vi "digital waveforms.vi"(11 "SD method in":T1 {"method array"."offset" format="%.2f"; "method array"."amplitude" format="%.2f"; "method array"."cycles/repeat period" min=1}) -> (2 "waveforms out":T2 format="%.2f", 3 "SD method out":T1 {"method array"."offset" format="%.2f"; "method array"."amplitude" format="%.2f"; "method array"."cycles/repeat period" min=1})   [LabVIEW 2010]
uses:
  SDMethod.ctl
  wavecluster.ctl
  <vilib>/Analysis/NI_AALBase.lvlib
panel:
  # "ticks"
  # "hz"
  # "ticks"
  # "ticks"
  # "volts"
  # "volts"
  # "ticks"
  # "hz"
  # "ticks"
  # "ticks"
  # "volts"
  # "volts"
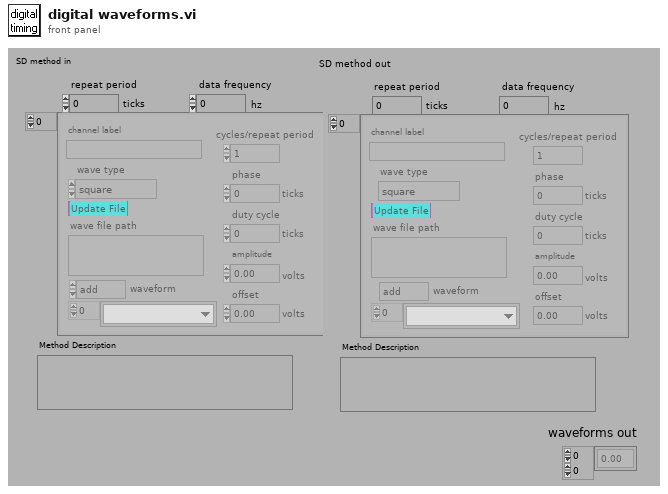
[diagram p1: front panel]
types:
  T1 = typedef "SDMethod.ctl" = cluster{"method array":cluster{"wave type":enum16{"off", "square", "sine", "triangle", "sawtooth", "from file", "wavemaker", "flume pump"}, "cycles/repeat period":u32, "phase":i32, "duty cycle":u32, "wave file path":path, "amplitude":dbl, "channel label":string, "Update":bool, "offset":dbl, " waveform":u16[], "Function":enum16{"add", "multiply"}}[], "Method Description":string, "data frequency":u32, "repeat period":u32}
  T2 = typedef "wavecluster.ctl" = sgl[][]
  T3 = cluster{"wave type":enum16{"off", "square", "sine", "triangle", "sawtooth", "from file", "wavemaker", "flume pump"}, "cycles/repeat period":u32, "phase":i32, "duty cycle":u32, "wave file path":path, "amplitude":dbl, "channel label":string, "Update":bool, "offset":dbl, " waveform":u16[], "Function":enum16{"add", "multiply"}}[]
  T4 = enum16{"off", "square", "sine", "triangle", "sawtooth", "from file", "wavemaker", "flume pump"}
  T5 = cluster{"wave type":enum16{"off", "square", "sine", "triangle", "sawtooth", "from file", "wavemaker", "flume pump"}, "cycles/repeat period":u32, "phase":i32, "duty cycle":u32, "wave file path":path, "amplitude":dbl, "channel label":string, "Update":bool, "offset":dbl, " waveform":u16[], "Function":enum16{"add", "multiply"}}
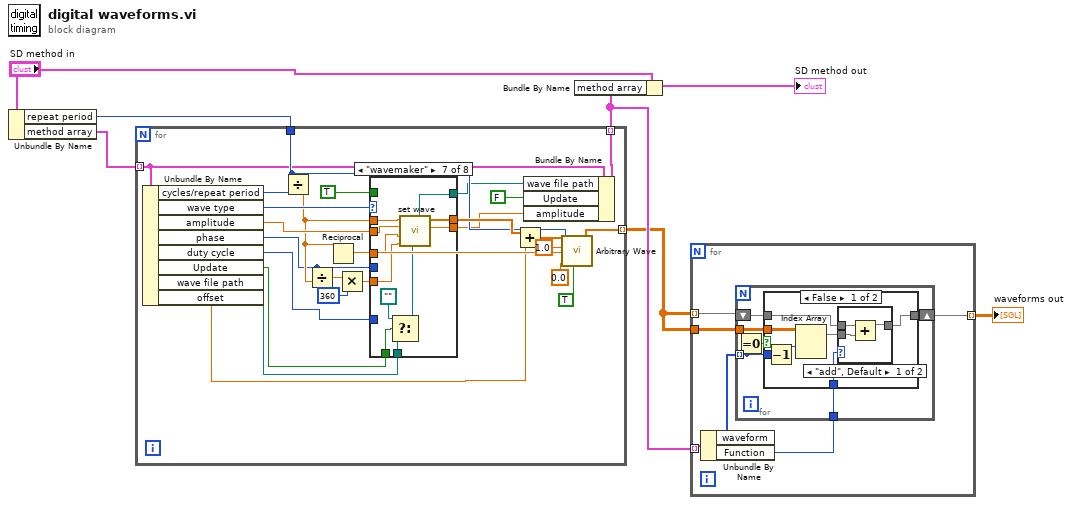
[diagram p0: block diagram]
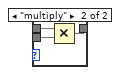
[diagram p2: hidden frame]
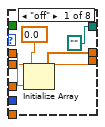
[diagram p4: hidden frame]
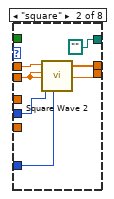
[diagram p5: hidden frame]
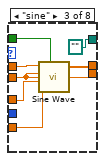
[diagram p6: hidden frame]
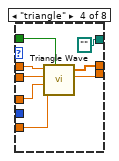
[diagram p7: hidden frame]
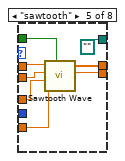
[diagram p8: hidden frame]
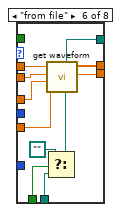
[diagram p9: hidden frame]
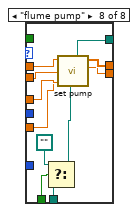
[diagram p10: hidden frame]
diagram:
  n1 = Unbundle By Name("SD method in") -> ("repeat period"=w5:u32, "method array"=w4:T3)
  n2 = for {
    tunnel: w4 -> [w16] mode=indexing
    tunnel: w5 -> [w20]
    tunnel: [w33] -> w2 mode=indexing
    tunnel: [w13] -> w3 mode=indexing
    n3 = Unbundle By Name(w16) -> ("cycles/repeat period"=w19:u32, "wave type"=w29:T4, "amplitude"=w21:dbl, "phase"=w10:i32, "duty cycle"=w11:u32, "Update"=w17:bool, "wave file path"=w12:path, "offset"=w8:dbl)
    n4 = Divide(x=w20, y=w19) -> (x/y=w18:dbl)
    n5 = Divide(x=w10, y=w18) -> (x/y=w27:dbl)
    n6 = Reciprocal(x=w18) -> (1/x=w30:dbl)
    n7 = Multiply(x=w27, y=u32 360) -> (x*y=w26:dbl)
    n8 = case shown="\"wavemaker\"" w29 {
      tunnel: w18 -> [w37 w44 w50 w57 w64 w70 w79 w90]
      tunnel: w21 -> [w34 w39 w45 w56 w59 w66 w77 w88]
      tunnel: w11 -> [_ w43 _ _ _ _ _ _]
      tunnel: w26 -> [_ _ w46 w52 w60 w67 w76 w87]
      tunnel: TRUE ("reset phase") -> [_ _ w51 w58 w65 _ _ _]
      tunnel: w30 -> [_ _ w49 w55 w63 w69 w78 w89]
      tunnel: [w36 w42 w48 w54 w62 w68 w81 w92] -> w22
      tunnel: w17 -> [_ _ _ _ _ w75 w83 w94]
      tunnel: [path "" path "" path "" path "" path "" w72 w86 w97] -> w15
      tunnel: w12 -> [_ _ _ _ _ w74 w85 w96]
      tunnel: w10 -> [_ w40 _ _ _ _ _ _]
      tunnel: [w34 w39 w45 w56 w59 w66 w80 w91] -> w9
      frame "off" {
        n9 = Initialize Array(0.0, w37) -> (w36:dbl[])
      }
      frame "square" {
        n10 = call "Square Wave 2.vi"("samples"=w44, "amplitude"=w39, "duty (ticks)"=w43, "phase ticks"=w40) -> ("Square Wave"=w42:dbl[])  [unwired: 3 in, 1 out]
      }
      frame "sine" {
        n11 = call <vilib>:"Sine Wave.vi"("samples"=w50, "amplitude"=w45, "frequency"=w49, "phase in"=w46, "reset phase"=w51) -> ("sine wave"=w48:dbl[])  [unwired: 2 out]
      }
      frame "triangle" {
        n12 = call <vilib>:"Triangle Wave.vi"("samples"=w57, "amplitude"=w56, "frequency"=w55, "phase in"=w52, "reset phase"=w58) -> ("triangle wave"=w54:dbl[])  [unwired: 2 out]
      }
      frame "sawtooth" {
        n13 = call <vilib>:"Sawtooth Wave.vi"("samples"=w64, "amplitude"=w59, "frequency"=w63, "phase in"=w60, "reset phase"=w65) -> ("sawtooth wave"=w62:dbl[])  [unwired: 2 out]
      }
      frame "from file" {
        n14 = Select(t=path "", s=w75, f=w74) -> (s? t:f=w71:path)
        n15 = call "get waveform.vi"("file path"=w71, "phase"=w67, "f"=w69, "amplitude"=w66, "samples"=w70) -> ("waveform"=w68:sgl[], "new file path"=w72:path)  [unwired: 4 in, 1 out]
      }
      frame "wavemaker" {
        n16 = Select(t=path "", s=w83, f=w85) -> (s? t:f=w82:path)
        n17 = call "set wave.vi"("file path"=w82, "phase"=w76, "f"=w78, "amplitude (volts) in"=w77, "samples"=w79) -> ("amplitude (volts)"=w80:dbl, "waveform"=w81:sgl[], "new file path"=w86:path)  [unwired: 4 in]
      }
      frame "flume pump" {
        n18 = Select(t=path "", s=w94, f=w96) -> (s? t:f=w93:path)
        n19 = call "set pump.vi"("file path"=w93, "phase"=w87, "f"=w89, "amplitude (volts) in"=w88, "samples"=w90) -> ("amplitude (volts)"=w91:dbl, "waveform"=w92:sgl[], "new file path"=w97:path)  [unwired: 4 in]
      }
    }
    n20 = Add(x=w22, y=w8) -> (x+y=w23:dbl[])
    n21 = Bundle By Name(cluster=w16, "wave file path"=w15, "Update"=FALSE, "amplitude"=w9) -> (w13:T5)
    n22 = call <vilib>:"Arbitrary Wave.vi"("reset phase"=TRUE, "Wave Table"=w23, "phase in"=0.0, "frequency"=w30, "amplitude"=1.0, "samples"=w20) -> ("arbitrary wave"=w33:dbl[])  [unwired: 1 in, 2 out]
  }
  n23 = Bundle By Name(cluster="SD method in", "method array"=w3) -> (→"SD method out":T1)
  n24 = for {
    tunnel: w2 -> [w102]
    tunnel: w3 -> [w103] mode=indexing
    tunnel: w2 -> [w101] mode=indexing
    tunnel: [w100] -> w1 mode=indexing
    n25 = Unbundle By Name(w103) -> ("waveform"=w99:u16[], "Function"=w98:enum16{"add", "multiply"})
    n26 = for {
      tunnel: w99 -> [w106] mode=indexing
      tunnel: w102 -> [w109]
      shift-right: [w107] -> w100
      shift-left: w101 -> [w108]
      tunnel: w98 -> [w104]
      n27 = Equal To 0?(x=w106) -> (x = 0?=w105:bool)
      n28 = case shown="False" w105 {
        tunnel: w109 -> [w116 _]
        tunnel: w106 -> [w115 _]
        tunnel: w108 -> [w113 w123]
        tunnel: [w112 w123] -> w107
        tunnel: w104 -> [w110 _]
        frame False {
          n29 = Decrement(x=w115) -> (x-1=w111:u16)
          n30 = Index Array(array=w116, index (row)=w111) -> (element=w114:dbl[])  [unwired: 1 in]
          n31 = case shown="\"add\", Default" w110 {
            tunnel: w114 -> [w119 w121]
            tunnel: w113 -> [w118 w122]
            tunnel: [w117 w120] -> w112
            frame "add", Default {
              n32 = Add(x=w118, y=w119) -> (x+y=w117:dbl[])
            }
            frame "multiply" {
              n33 = Multiply(x=w122, y=w121) -> (x*y=w120:dbl[])
            }
          }
        }
        frame True {
        }
      }
    }
  }
  "waveforms out" <- w1
